vi "Get Channel Name.vi"(8 "error in (no error)":errorcluster, 10 "Channel Index (1)":i32=1, 11 "CS++Fgen in":refnum<class "CS++Fgen.lvclass">) -> (0 "error out":errorcluster, 2 "Channel Name":string, 3 "CS++Fgen out":refnum<class "CS++Fgen.lvclass">)   [LabVIEW 2015, in "CS++Fgen.lvlib" / "CS++Fgen.lvclass"]
doc: "This VI returns the highest-level channel name that corresponds to the specific driver channel string that is in the channel table at an index you specify."
uses:
  CS++Fgen.lvclass
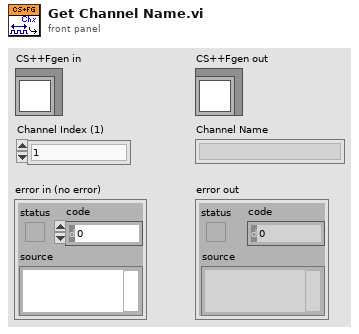
[diagram p1: front panel]
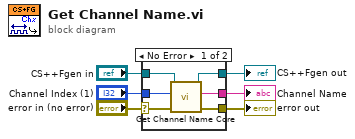
[diagram p0: block diagram]
diagram:
  n1 = case shown="No Error" "error in (no error)" {
    selector: "error in (no error)" -> [w9 w14]
    tunnel: [w7 w14] -> w5
    tunnel: [w11 w13] -> w3
    tunnel: "CS++Fgen in" -> [w12 w13]
    tunnel: "Channel Index (1)" -> [w10 _]
    tunnel: [w8 _] -> w1
    frame No Error {
      n2 = call-dynamic "Get Channel Name Core.vi"("error in (no error)"=w9, "Channel Index (1)"=w10, "CS++Fgen in"=w12) -> ("error out"=w7:errorcluster, "Channel Name"=w8:string, "CS++Fgen out"=w11:refnum<class "CS++Fgen.lvclass">)  [unwired: 6 in]
    }
    frame Error {
    }
  }
  "error out" <- w5
  "CS++Fgen out" <- w3
  "Channel Name" <- w1
